vi "AK-LNI Antwortstring teilen_ALT.vi"(11 "Antwortstring":string) -> (3 "Empfangsdaten":string[](array[string]))   [LabVIEW 2020, in "Linearisierung v2.lvlib" / "Gasteiler.lvlib" / "AK Komm Gasteiler.lvlib" / "Alter Gasteiler.lvlib"]
doc: "Trennt den Antwortstring, in dem jedes Argument mit einem Leerzeichen beginnt, in die einzelnen Argumente auf. Die Empfangsdaten enthalten in jedem Arrayelement ein Argument als String."
uses:
  Alter Gasteiler.lvlib
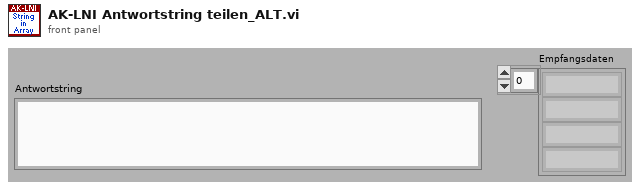
[diagram p1: front panel]
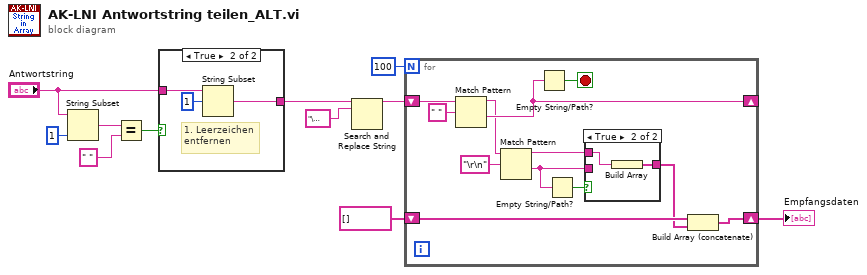
[diagram p0: block diagram]
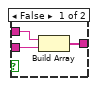
[diagram p2: hidden frame]
diagram:
  n1 = String Subset(string="Antwortstring", length (rest)=1 ("Länge (Rest)")) -> (substring=w10:string)  [unwired: 1 in]
  n2 = Equal?(x=w10, y=" ") -> (x = y?=w8:bool)
  n3 = case shown="True" w8 {
    tunnel: "Antwortstring" -> [w12 w15]
    tunnel: [w12 w13] -> w3
    frame False {
    }
    frame True {
      # "1. Leerzeichen\nentfernen"
      n4 = String Subset(string=w15, offset (0)=1 ("Länge (Rest)")) -> (substring=w13:string)  [unwired: 1 in]
    }
  }
  n5 = Search and Replace String(input string=w3, search string="\u0003" ("Such-String")) -> (result string=w2:string)  [unwired: 6 in, 3 out]
  n6 = for {
    N: 100 -> [_]
    shift-right: [w23] -> _
    shift-left: w2 -> [w27]
    shift-right: [w24] -> w1
    shift-left: string[] [] -> [w25]
    stop <- w22 stop-if-true
    n7 = Match Pattern(string=w27, regular expression=" " ("Trennzeichen (Tabulator)")) -> (before substring=w19:string, after substring=w23:string)  [unwired: 1 in, 2 out]
    n8 = Match Pattern(string=w19, regular expression="\r\n" ("Trennzeichen (Tabulator)")) -> (before substring=w21:string, after substring=w18:string)  [unwired: 1 in, 2 out]
    n9 = Empty String/Path?(string/path=w23) -> (empty?=w22:bool)
    n10 = Empty String/Path?(string/path=w18) -> (empty?=w17:bool)
    n11 = case shown="True" w17 {
      tunnel: w18 -> [w30 _]
      tunnel: w21 -> [w29 w32]
      tunnel: [w28 w31] -> w16
      frame False {
        n12 = Build Array(w29, w30) -> (w28:string[])
      }
      frame True {
        n13 = Build Array(w32) -> (w31:string[])
      }
    }
    n14 = Build Array (concatenate)(w25, w16) -> (w24:string[])
  }
  "Empfangsdaten" <- w1
